vi "Eval Func at Sampling Pnts.vi"(6 "variable output":string, 7 "variable input":string, 8 "error in (no error)":errorcluster, 9 "formula":string, 10 "lower limit":dbl, 11 "upper limit":dbl) -> (0 "error out":errorcluster, 2 "Sampling points (7-order)":dbl[](array[numeric]), 3 "Function Evaluations (7 and 4 pts)":dbl[](array[numeric]))   [LabVIEW 2010, in "NI_AALPro.lvlib"]
uses:
  NI_AALPro.lvlib
  NI_Gmath.lvlib
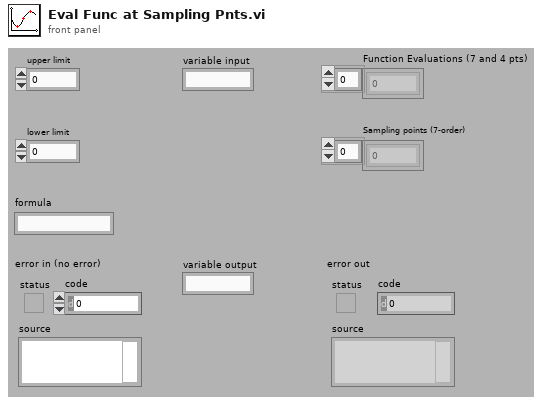
[diagram p1: front panel]
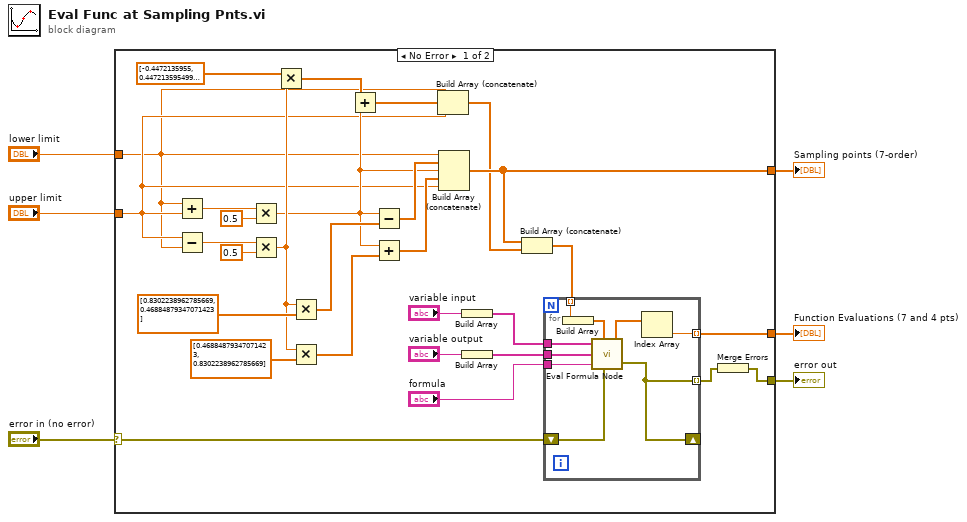
[diagram p0: block diagram]
diagram:
  n1 = case shown="No Error" "error in (no error)" {
    selector: "error in (no error)" -> [w21 w45]
    tunnel: [w12 _] -> w6
    tunnel: [w27 _] -> w5
    tunnel: [w7 w45] -> w4
    tunnel: "lower limit" -> [w9 _]
    tunnel: "upper limit" -> [w14 _]
    frame No Error {
      n2 = Add(x=w9, y=w14) -> (x+y=w25:dbl)
      n3 = Subtract(x=w14, y=w9) -> (x-y=w23:dbl)
      n4 = Multiply(x=w25, y=0.5) -> (x*y=w16:dbl)
      n5 = Multiply(x=w23, y=0.5) -> (x*y=w18:dbl)
      n6 = Multiply(x=dbl[] [-0.4472135955, 0.4472135954999579] ("appended array"), y=w18) -> (x*y=w17:dbl[])
      n7 = Multiply(x=w18, y=dbl[] [0.8302238962785669, 0.46884879347071423] ("appended array")) -> (x*y=w31:dbl[])
      n8 = Multiply(x=w18, y=dbl[] [0.46884879347071423, 0.8302238962785669] ("appended array")) -> (x*y=w30:dbl[])
      n9 = Add(x=w17, y=w16) -> (x+y=w15:dbl[])
      n10 = Subtract(x=w16, y=w31) -> (x-y=w29:dbl[])
      n11 = Add(x=w16, y=w30) -> (x+y=w28:dbl[])
      n12 = Build Array (concatenate)(w9, w15, w14) -> (w11:dbl[])
      n13 = Build Array (concatenate)(w9, w29, w16, w28, w14) -> (w12:dbl[])
      n14 = Build Array("variable input") -> (w34:string[])
      n15 = Build Array("variable output") -> (w32:string[])
      n16 = Build Array (concatenate)(w12, w11) -> (w13:dbl[])
      n17 = for {
        tunnel: "formula" -> [w44]
        tunnel: w34 -> [w43]
        tunnel: w32 -> [w42]
        tunnel: w13 -> [w41] mode=indexing
        tunnel: [w40] -> w27 mode=indexing
        tunnel: [w36] -> w8 mode=indexing
        shift-right: [w36] -> _
        shift-left: w21 -> [w37]
        n18 = Build Array(w41) -> (w39:dbl[])
        n19 = call "Eval Formula Node.vi"("Variables Input"=w43, "Input Values"=w39, "Variables Output"=w42, "formula"=w44, "error in (no error)"=w37) -> ("Output Values"=w38:dbl[], "error out"=w36:errorcluster)
        n20 = Index Array(array=w38) -> (element=w40:dbl)  [unwired: 1 in]
      }
      n21 = Merge Errors(w8) -> (w7:errorcluster)
    }
    frame Error {
    }
  }
  "Sampling points (7-order)" <- w6
  "Function Evaluations (7 and 4 pts)" <- w5
  "error out" <- w4
